vi "Create Test Reporter Configuration.vi"() -> (2 "String":string, 3 "ResultProcessor Config out":refnum<class "ResultProcessor Config.lvclass">)   [LabVIEW 2015, in "Sequencer Module tests.lvlib"]
uses:
  Sequencer Module tests.lvlib
  classes/Result Processor/Config/ResultProcessor Config.lvclass
  classes/Report/On-The-Fly/Config/OnTheFlyReport Config.lvclass
  classes/Report Formatters/csv/Config/csv-formatter Config.lvclass
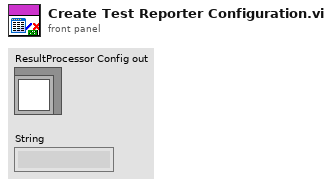
[diagram p1: front panel]
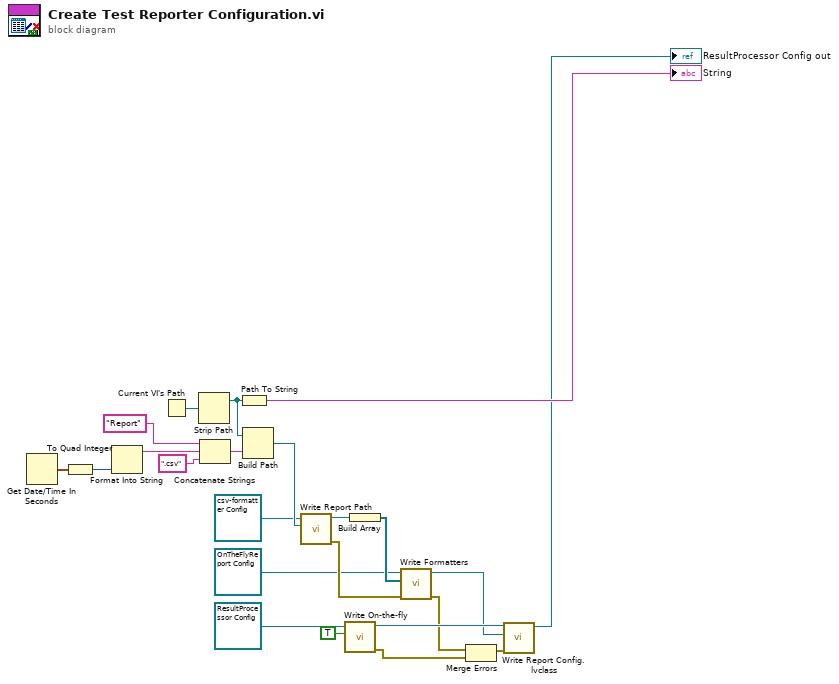
[diagram p0: block diagram]
diagram:
  n1 = Get Date/Time In Seconds() -> (seconds since 1Jan1904=w20:timestamp)
  n2 = To Quad Integer(1:w20) -> (0:w18:i64)
  n3 = Format Into String(w18) -> (resulting string=w19:string)  [unwired: 3 in, 1 out]
  n4 = Current VI's Path() -> (path=w8:path)
  n5 = Strip Path(path=w8) -> (stripped path=w22:path)  [unwired: 1 out]
  n6 = Concatenate Strings("Report" ("string"), w19, ".csv" ("string")) -> (w11:string)
  n7 = Path To String(path=w22) -> (string=→"String":string)
  n8 = Build Path(base path=w22, name or relative path=w11) -> (appended path=w21:path)
  n9 = call-dynamic "Write Report Path.vi"("Report Path"=w21, "csv-formatter Config in"=refnum<class "csv-formatter Config.lvclass"> refnum ("csv-formatter Config.lvclass")) -> ("error out"=w12:errorcluster, "csv-formatter Config out"=w7:refnum<class "csv-formatter Config.lvclass">)  [unwired: 8 in]
  n10 = call-dynamic "Write On-the-fly.vi"("On-the-fly?"=TRUE, "ResultProcessor Config in"=refnum<class "ResultProcessor Config.lvclass"> refnum) -> ("error out"=w17:errorcluster, "ResultProcessor Config out"=w14:refnum<class "ResultProcessor Config.lvclass">)  [unwired: 8 in]
  n11 = Build Array(w7) -> (w3:refnum<class "csv-formatter Config.lvclass">[])
  n12 = call-dynamic "Write Formatters.vi"("error in (no error)"=w12, "Formatters"=w3, "OnTheFlyReport Config in"=refnum<class "OnTheFlyReport Config.lvclass"> refnum ("OnTheFlyReport Config.lvclass")) -> ("error out"=w4:errorcluster, "OnTheFlyReport Config out"=w2:refnum<class "OnTheFlyReport Config.lvclass">)  [unwired: 7 in]
  n13 = Merge Errors(w4, w17) -> (w16:errorcluster)
  n14 = call-dynamic "Write Report Config.lvclass.vi"("error in (no error)"=w16, "Report Config.lvclass"=w2, "ResultProcessor Config in"=w14) -> ("ResultProcessor Config out"=→"ResultProcessor Config out":refnum<class "ResultProcessor Config.lvclass">)  [unwired: 7 in, 1 out]
